vi "Last Ack Creator Queue.vi"(10 "Queue":refnum<class "Queue.lvclass">, 11 "Template Event in":refnum<class "Template Event.lvclass">) -> (3 "Template Event out":refnum<class "Template Event.lvclass">)   [LabVIEW 2021, in "_Template.lvlib" / "Templates.lvlib" / "Template Event.lvlib" / "Template Event.lvclass"]
uses:
  Template Event.lvclass
  Template Event.lvclass/Template Event.ctl
  <vilib>/jettl/jettl/jettl/Queue/Queue.lvclass
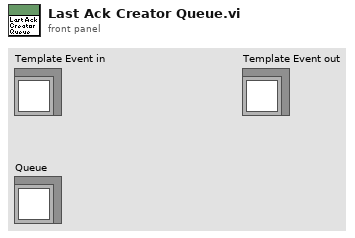
[diagram p1: front panel]
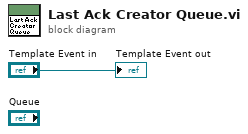
[diagram p0: block diagram]
diagram:
  "Template Event out" <- "Template Event in"
